vi "10-5-5-2.vi"() -> ()   [LabVIEW 2025]
uses:
  <vilib>/Platform/TimedLoop/XDataNode/timing_clust.ctl
  <vilib>/Platform/TimedLoop/XDataNode/nitl_modes.ctl
  <vilib>/Platform/TimedLoop/XDataNode/wakeup.ctl
  <vilib>/rvi/Emulation/niFpgaSctlEmulationGetInTimedLoop.vi
  <vilib>/rvi/Emulation/niFpgaEmulationReportErrorSimple.vi
  <vilib>/rvi/Emulation/niFpgaGetClockAttributes.vi
  <vilib>/rvi/Emulation/niFpgaCriticalErrorInLSC.vi
  <vilib>/rvi/linearAlgebra/MatrixMultiply/simVIs/SubVI/nifxpla_MatrixMultiply_SimMatrixSizes.vi
  <vilib>/rvi/linearAlgebra/MatrixMultiply/simVIs/SubVI/nifxpla_MatrixMultiply_Sim4WireAdapterVector.vi
  <vilib>/rvi/linearAlgebra/MatrixMultiply/simVIs/SubVI/nifxpla_MatrixMultiply_SimFrameHandShake.vi
  <vilib>/rvi/linearAlgebra/MatrixMultiply/simVIs/SubVI/nifxpla_MatrixMultiply_SimEndlessCounter.vi
  <vilib>/rvi/linearAlgebra/MatrixMultiply/simVIs/SubVI/nifxpla_MatrixMultiply_SimVectorDataBuffer.vi
  <vilib>/rvi/ClientSDK/Core/DevComputerLib/Private/Multiply(dfxp64).vi
  <vilib>/rvi/ClientSDK/Core/DevComputerLib/Private/Dfxp128ToDfxp256.vi
  <vilib>/rvi/ClientSDK/Core/DevComputerLib/Private/Add(dfxp256).vi
  <vilib>/rvi/ClientSDK/Core/DevComputerLib/Private/Subtract(dfxp256).vi
  <vilib>/rvi/ClientSDK/Core/DevComputerLib/Private/ToDfxp64(dfxp256).vi
  <vilib>/platform/TimedLoop/XDataNode/XDataNode.xnode
  <vilib>/rvi/linearAlgebra/MatrixMultiply/XNode/nifxpla_MatrixMultiply.xnode
  <vilib>/rvi/linearAlgebra/MatrixMultiply/simVIs/nifxpla_MatrixMultiply_SimTemplateEinEout.vi
  <vilib>/rvi/linearAlgebra/MatrixMultiply/simVIs/nifxpla_MatrixMultiply_SimTemplateEinVout.vi
  <vilib>/rvi/linearAlgebra/MatrixMultiply/simVIs/nifxpla_MatrixMultiply_SimTemplateVinEout.vi
  <vilib>/rvi/linearAlgebra/MatrixMultiply/simVIs/nifxpla_MatrixMultiply_SimTemplateVinVout.vi
  <vilib>/Platform/TimedLoop/XDataNode/XDNodeRunTimeDep.lvlib
panel:
  out "Latency":u32
  out "C3+B":fxp<+/-,33,17>[](array[numeric])
  out "C3":fxp<+/-,32,16>[](array[numeric])
  out "Cycle Count 3":i32
  out "C2+B":fxp<+/-,33,17>[](array[numeric])
  out "C2":fxp<+/-,32,16>[](array[numeric])
  out "Cycle Count 2":i32
  out "C1+B":fxp<+/-,33,17>[](array[numeric])
  out "C1":fxp<+/-,32,16>[](array[numeric])
  out "Cycle Count":i32
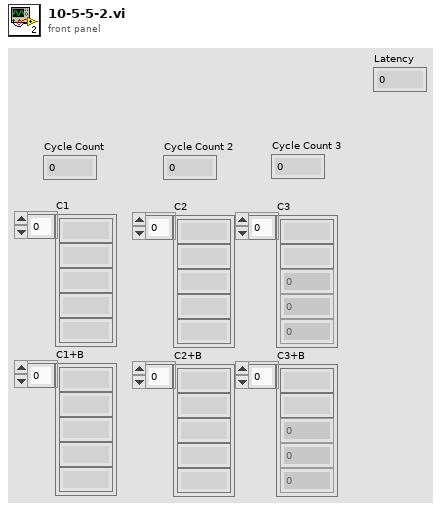
[diagram p1: front panel]
types:
  T1 = typedef "XDNodeRunTimeDep.lvlib/timing_clust.ctl" = cluster{"Expected End [f-1]":u64, "Actual End [f-1]":u64, "Finished Late? [f-1]":bool, "Expected End [i-1]":u64, "Actual End [i-1]":u64, "Finished Late? [i-1]":bool, "Expected Start [i]":u64, "Actual Start [i]":u64, "Expected Start [f]":u64, "Actual Start [f]":u64, "Source Name":string, "Structure Name":string, "Period":i64, "Deadline":i64, "Offset":i64, "Start":i64, "Priority":i32, "Timeout":i32, "Mode":T2, "Wakeup Reason":T3, "Error":errorcluster, "Source Type":string, "Secondary Source Type":string, "Global End Time":u64, "Global Start Time":u64, "Frame Duration":u64, "Iteration Duration":u64, "Assigned CPU":i32, "I/O Scan Engine Mode":u32}
  T2 = typedef "XDNodeRunTimeDep.lvlib/nitl_modes.ctl" = enum32{"No Change", "Process missed periods, maintain original phase", "Discard missed periods, maintain original phase", "Process missed periods, ignore original phase", "Discard missed periods, ignore original phase"}
  T3 = typedef "XDNodeRunTimeDep.lvlib/wakeup.ctl" = enum32{"Normal", "Aborted", "Asynchronous wakeup", "Timing source error", "Timed loop error", "Timeout"}
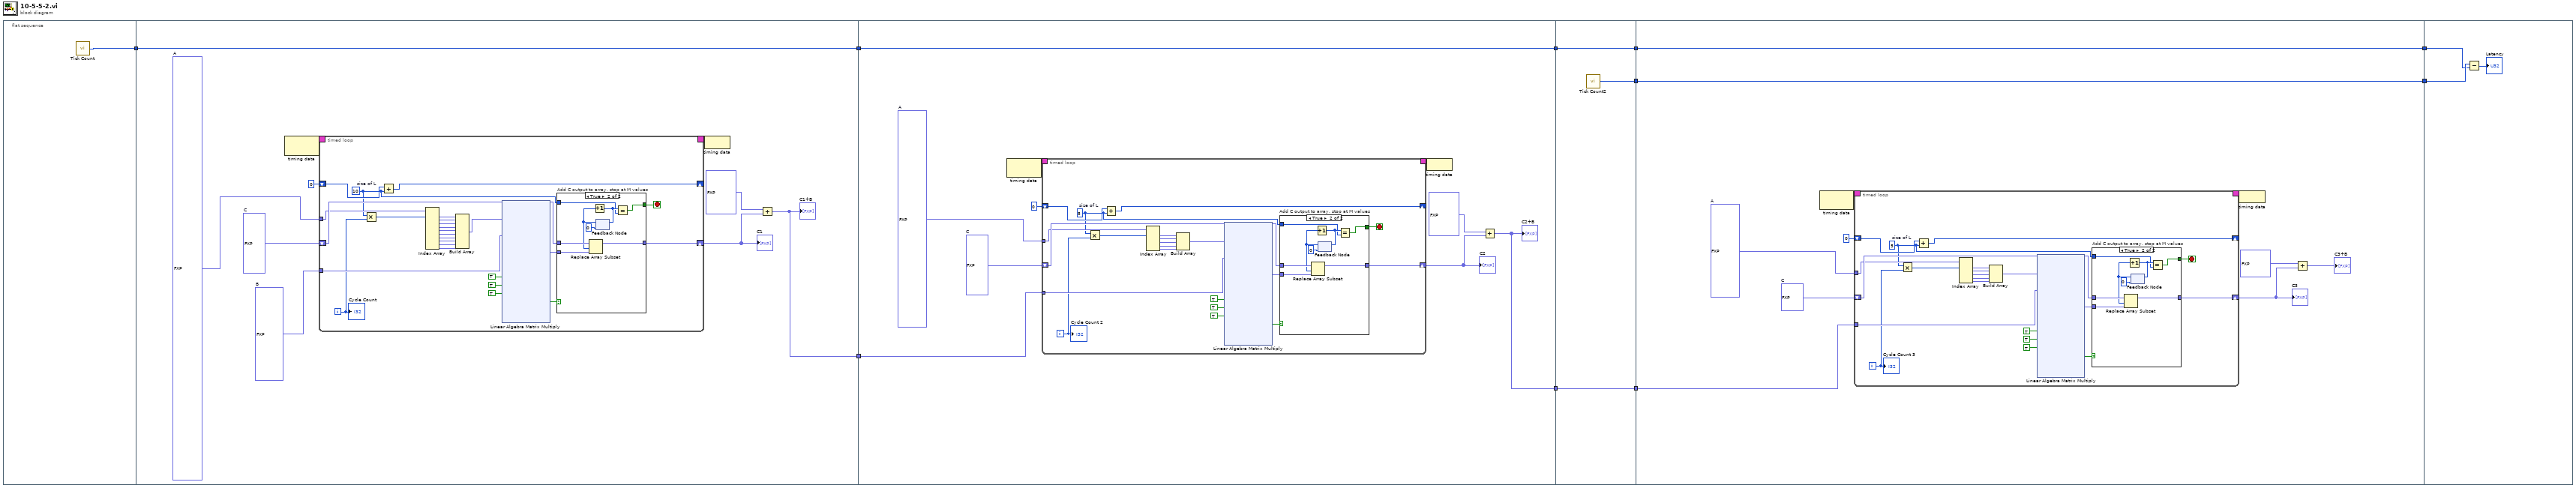
[diagram p0: block diagram]
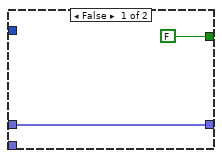
[diagram p2: hidden frame]
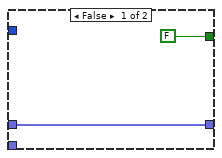
[diagram p3: hidden frame]
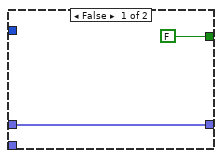
[diagram p4: hidden frame]
diagram:
  n1 = flat-sequence {
    tunnel: [w11] -> w8
    tunnel: [w13] -> w10
    tunnel: [w12] -> w9
    tunnel: w8 -> [w12]
    tunnel: w10 -> [w64]
    tunnel: [w63] -> w6
    tunnel: w9 -> [w62]
    tunnel: [w62] -> w4
    tunnel: w6 -> [w109]
    tunnel: [w109] -> w5
    tunnel: w4 -> [w108]
    tunnel: [w108] -> w3
    tunnel: [w107] -> w1
    tunnel: w5 -> [w112]
    tunnel: w3 -> [w111]
    tunnel: [w111] -> w7
    tunnel: [w110] -> w2
    tunnel: w1 -> [w110]
    tunnel: w7 -> [w157]
    tunnel: w2 -> [w158]
    frame #0 {
      n2 = call "Tick Count"() -> ("Tick Count(Ticks)"=w11:u32)
    }
    frame #1 {
      w17 = fxp<+/-,32,16>[] [1.0, 2.0, 3.0, 4.0, 5.0, 1.0, 2.0, 3.0, 4.0, 5.0, 1.0, 2.0, 3.0, 4.0, 5.0, 1.0, 2.0, 3.0, 4.0, 5.0, 1.0, 2.0, 3.0, 4.0, 5.0, 1.0, 2.0, 3.0, 4.0, 5.0, 1.0, 2.0, 3.0, 4.0, 5.0, 1.0, 2.0, 3.0, 4.0, 5.0, 1.0, 2.0, 3.0, 4.0, 5.0, 1.0, 2.0, 3.0, 4.0, 5.0]  # A
      w18 = fxp<+/-,32,16>[] [1.0, 2.0, 3.0, 4.0, 5.0, 1.0, 2.0, 3.0, 4.0, 5.0]  # B
      w19 = fxp<+/-,32,16>[] [0.0, 0.0, 0.0, 0.0, 0.0]  # C
      n3 = node-c288() -> (w21:T1)  [unwired: 1 in]
      n4 = timed-loop {
        timing: w21 -> [_]
        timing-out: [_] -> w20
        shift-right: [w46] -> w15
        shift-left: w19 -> [w45]
        tunnel: w18 -> [w42]
        tunnel: w17 -> [w25]
        shift-right: [w38] -> _
        shift-left: 0 ("length") -> [w39]
        i -> [w24]
        stop <- w44 stop-if-true
        w23 = 10  # size of L
        n5 = Multiply(x=w23, y=w24) -> (x*y=w36:i32)
        n6 = Add(x=w39, y=w23) -> (x+y=w38:i32)
        n7 = Index Array(array=w25, index #1=w36) -> (element #1=w35:fxp<+/-,32,16>, element #2=w34:fxp<+/-,32,16>, element #3=w33:fxp<+/-,32,16>, element #4=w32:fxp<+/-,32,16>, element #5=w31:fxp<+/-,32,16>, element #6=w30:fxp<+/-,32,16>, element #7=w29:fxp<+/-,32,16>, element #8=w28:fxp<+/-,32,16>, element #9=w27:fxp<+/-,32,16>, element #10=w26:fxp<+/-,32,16>)  [unwired: 9 in]
        n8 = Build Array(w35, w34, w33, w32, w31, w30, w29, w28, w27, w26) -> (w22:fxp<+/-,32,16>[])
        n9 = xnode ("Linear Algebra Matrix Multiply")("ar"=w22, "br"=w42, "a valid"=TRUE, "b valid"=TRUE, "ready for output (T)"=TRUE) -> ("cr"=w41:fxp<+/-,64,36>[], "output valid"=w37:bool)  [unwired: 2 in, 4 out]
        n10 = case "Add C output to array, stop at M values" shown="True" w37 {
          tunnel: w41 -> [_ w53]
          tunnel: [w49 w56] -> w46
          tunnel: w45 -> [w49 w57]
          tunnel: [FALSE w54] -> w44
          tunnel: w23 -> [_ w50]
          frame False {
          }
          frame True {
            n11 = feedback #1(0 ("x")) -> (w52:i32)
            n12 = Replace Array Subset(array=w57, new element=w53, index=w52) -> (w56:fxp<+/-,32,16>[])
            n13 = Increment(x=w52) -> (x+1=w51:i32)
            n14 = feedback-in #1(w51) -> ()
            n15 = Equal?(x=w51, y=w50) -> (x = y?=w54:bool)
          }
        }
        "Cycle Count" <- w24
      }
      "C1" <- w15
      n16 = node-c288(w20) -> ()
      n17 = Add(x=fxp<+/-,32,16>[] [0.5, 0.5, 0.5, 0.5, 0.5], y=w15) -> (x+y=w13:fxp<+/-,33,17>[])
      "C1+B" <- w13
    }
    frame #2 {
      w68 = fxp<+/-,32,16>[] [1.0, 2.0, 3.0, 4.0, 5.0, 1.0, 2.0, 3.0, 4.0, 5.0, 1.0, 2.0, 3.0, 4.0, 5.0, 1.0, 2.0, 3.0, 4.0, 5.0, 1.0, 2.0, 3.0, 4.0, 5.0]  # A
      w69 = fxp<+/-,32,16>[] [0.0, 0.0, 0.0, 0.0, 0.0]  # C
      n18 = node-c288() -> (w71:T1)  [unwired: 1 in]
      n19 = timed-loop {
        timing: w71 -> [_]
        timing-out: [_] -> w70
        shift-right: [w91] -> w66
        shift-left: w69 -> [w90]
        tunnel: w64 -> [w87]
        tunnel: w68 -> [w75]
        shift-right: [w83] -> _
        shift-left: 0 ("length") -> [w84]
        i -> [w74]
        stop <- w89 stop-if-true
        w73 = 5  # size of L
        n20 = Multiply(x=w73, y=w74) -> (x*y=w81:i32)
        n21 = Add(x=w84, y=w73) -> (x+y=w83:i32)
        n22 = Index Array(array=w75, index #1=w81) -> (element #1=w80:fxp<+/-,32,16>, element #2=w79:fxp<+/-,32,16>, element #3=w78:fxp<+/-,32,16>, element #4=w77:fxp<+/-,32,16>, element #5=w76:fxp<+/-,32,16>)  [unwired: 4 in]
        n23 = Build Array(w80, w79, w78, w77, w76) -> (w72:fxp<+/-,32,16>[])
        n24 = xnode ("Linear Algebra Matrix Multiply")("ar"=w72, "br"=w87, "a valid"=TRUE, "b valid"=TRUE, "ready for output (T)"=TRUE) -> ("cr"=w86:fxp<+/-,64,36>[], "output valid"=w82:bool)  [unwired: 2 in, 4 out]
        n25 = case "Add C output to array, stop at M values" shown="True" w82 {
          tunnel: w86 -> [_ w98]
          tunnel: [w94 w101] -> w91
          tunnel: w90 -> [w94 w102]
          tunnel: [FALSE w99] -> w89
          tunnel: w73 -> [_ w95]
          frame False {
          }
          frame True {
            n26 = feedback #2(0 ("x")) -> (w97:i32)
            n27 = Replace Array Subset(array=w102, new element=w98, index=w97) -> (w101:fxp<+/-,32,16>[])
            n28 = Increment(x=w97) -> (x+1=w96:i32)
            n29 = feedback-in #2(w96) -> ()
            n30 = Equal?(x=w96, y=w95) -> (x = y?=w99:bool)
          }
        }
        "Cycle Count 2" <- w74
      }
      "C2" <- w66
      n31 = node-c288(w70) -> ()
      n32 = Add(x=fxp<+/-,32,16>[] [0.5, 0.5, 0.5, 0.5, 0.5], y=w66) -> (x+y=w63:fxp<+/-,33,17>[])
      "C2+B" <- w63
    }
    frame #3 {
      n33 = call "Tick Count2"() -> ("Tick Count(Ticks)"=w107:u32)
    }
    frame #4 {
      w117 = fxp<+/-,32,16>[] [2.0, 2.0, 2.0, 2.0, 2.0, 2.0, 2.0, 2.0, 2.0, 2.0]  # A
      w118 = fxp<+/-,32,16>[] [0.0, 0.0]  # C
      n34 = node-c288() -> (w120:T1)  [unwired: 1 in]
      n35 = timed-loop {
        timing: w120 -> [_]
        timing-out: [_] -> w119
        shift-right: [w140] -> w115
        shift-left: w118 -> [w139]
        tunnel: w112 -> [w136]
        tunnel: w117 -> [w124]
        shift-right: [w132] -> _
        shift-left: 0 ("length") -> [w133]
        i -> [w123]
        stop <- w138 stop-if-true
        w122 = 5  # size of L
        n36 = Multiply(x=w122, y=w123) -> (x*y=w130:i32)
        n37 = Add(x=w133, y=w122) -> (x+y=w132:i32)
        n38 = Index Array(array=w124, index #1=w130) -> (element #1=w129:fxp<+/-,32,16>, element #2=w128:fxp<+/-,32,16>, element #3=w127:fxp<+/-,32,16>, element #4=w126:fxp<+/-,32,16>, element #5=w125:fxp<+/-,32,16>)  [unwired: 4 in]
        n39 = Build Array(w129, w128, w127, w126, w125) -> (w121:fxp<+/-,32,16>[])
        n40 = xnode ("Linear Algebra Matrix Multiply")("ar"=w121, "br"=w136, "a valid"=TRUE, "b valid"=TRUE, "ready for output (T)"=TRUE) -> ("cr"=w135:fxp<+/-,64,36>[], "output valid"=w131:bool)  [unwired: 2 in, 4 out]
        n41 = case "Add C output to array, stop at M values" shown="True" w131 {
          tunnel: w135 -> [_ w147]
          tunnel: [w143 w150] -> w140
          tunnel: w139 -> [w143 w151]
          tunnel: [FALSE w148] -> w138
          tunnel: w122 -> [_ w144]
          frame False {
          }
          frame True {
            n42 = feedback #3(0 ("x")) -> (w146:i32)
            n43 = Replace Array Subset(array=w151, new element=w147, index=w146) -> (w150:fxp<+/-,32,16>[])
            n44 = Increment(x=w146) -> (x+1=w145:i32)
            n45 = feedback-in #3(w145) -> ()
            n46 = Equal?(x=w145, y=w144) -> (x = y?=w148:bool)
          }
        }
        "Cycle Count 3" <- w123
      }
      "C3" <- w115
      n47 = node-c288(w119) -> ()
      n48 = Add(x=fxp<+/-,32,16>[] [0.5, 0.5], y=w115) -> (x+y=→"C3+B":fxp<+/-,33,17>[])
    }
    frame #5 {
      n49 = Subtract(x=w158, y=w157) -> (x-y=→"Latency":u32)
    }
  }
